vi "SwrvLinAlg XY Relative to Robot.vi"(8 "x,y movement vector":dbl[](array[numeric]), 11 "Theta":dbl) -> (0 "A x Vector":dbl[](array[numeric]), 3 "Rotation Matrix by Theta":T1)   [LabVIEW 2017]
uses:
  <vilib>/Analysis/Matrix/Datatypes/RealMatrix.ctl
  <vilib>/Analysis/baseanly.llb/A x Vector.vi
  <vilib>/Analysis/NI_AALBase.lvlib
  <vilib>/Analysis/Matrix/NI_Matrix.lvlib
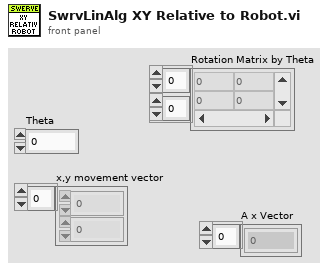
[diagram p1: front panel]
types:
  T1 = typedef "NI_Matrix.lvlib/RealMatrix.ctl" = dbl[][]
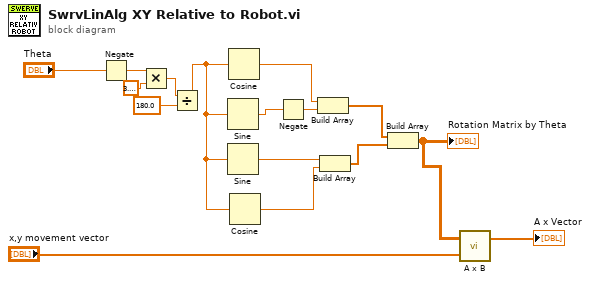
[diagram p0: block diagram]
diagram:
  n1 = Negate(x="Theta") -> (-x=w3:dbl)
  n2 = Multiply(x=w3, y=3.141592653589793) -> (x*y=w13:dbl)
  n3 = Divide(x=w13, y=180.0) -> (x/y=w11:dbl)
  n4 = Sine(x=w11) -> (sin(x)=w2:dbl)
  n5 = Sine(x=w11) -> (sin(x)=w7:dbl)
  n6 = Cosine(x=w11) -> (cos(x)=w5:dbl)
  n7 = Cosine(x=w11) -> (cos(x)=w8:dbl)
  n8 = Negate(x=w2) -> (-x=w1:dbl)
  n9 = Build Array(w5, w1) -> (w6:dbl[])
  n10 = Build Array(w7, w8) -> (w9:dbl[])
  n11 = Build Array(w6, w9) -> (w10:T1)
  "Rotation Matrix by Theta" <- w10
  n12 = call-poly <vilib>:"A x B.vi"("Vector"="x,y movement vector", "A"=w10) -> ("A x Vector"=→"A x Vector":dbl[])  [unwired: 1 out]
